vi "run stats.vi"(10 "percentiles":dbl[](array[numeric]), 11 "Data":dbl[](array[numeric])) -> (3 "stats out":T1)   [LabVIEW 2014]
uses:
  <vilib>/gmath/statdist.llb/st_Percentiles (scalar).vi
  <vilib>/Analysis/NI_AALBase.lvlib
  <vilib>/gmath/NI_Gmath.lvlib
  <vilib>/Analysis/NI_AALPro.lvlib
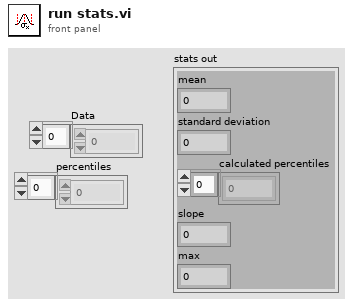
[diagram p1: front panel]
types:
  T1 = cluster{"mean":dbl, "standard deviation":dbl, "calculated percentiles":dbl[], "slope":dbl, "max":dbl}
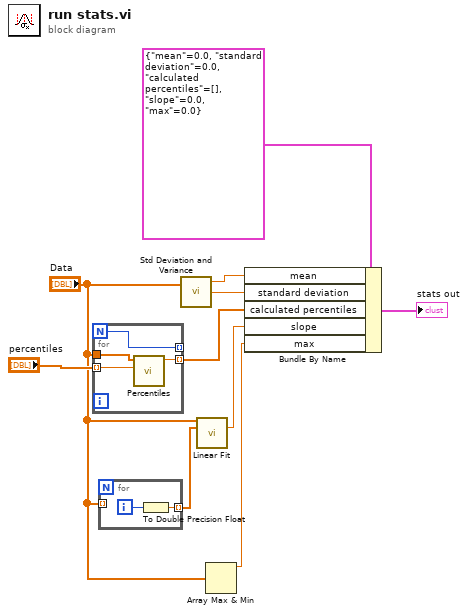
[diagram p0: block diagram]
diagram:
  n1 = for {
    N -> [w13]
    tunnel: [w14] -> w8 mode=indexing
    tunnel: [w13] -> _ mode=indexing
    tunnel: "Data" -> [w12]
    tunnel: "percentiles" -> [w11] mode=indexing
    n2 = call-poly <vilib>:"Percentiles.vi"("p"=w11, "x array"=w12) -> ("percentile"=w14:dbl)  [unwired: 8 in, 1 out]
  }
  n3 = for {
    tunnel: [w15] -> w6 mode=indexing
    tunnel: "Data" -> [_] mode=indexing
    i -> [w16]
    n4 = To Double Precision Float(number=w16) -> (double precision float=w15:dbl)
  }
  n5 = call <vilib>:"Std Deviation and Variance.vi"("X"="Data") -> ("mean"=w10:dbl, "standard deviation"=w9:dbl)  [unwired: 1 in, 1 out]
  n6 = call <vilib>:"Linear Fit.vi"("Y"="Data", "X"=w6) -> ("slope"=w4:dbl)  [unwired: 9 in, 4 out]
  n7 = Array Max & Min(array="Data") -> (max value=w2:dbl)  [unwired: 3 out]
  n8 = Bundle By Name(cluster=T1 {"mean"=0.0, "standard deviation"=0.0, "calculated percentiles"=[], "slope"=0.0, "max"=0.0} ("stats out"), "mean"=w10, "standard deviation"=w9, "calculated percentiles"=w8, "slope"=w4, "max"=w2) -> (→"stats out":T1)
